vi "PLAN IN FEEDING SCREEN.vi"(6 "LOOP DATA IN":T1, 7 "error IN":errorcluster, 10 "PLAN In":string[][](array[string])) -> (0 "error out":errorcluster, 1 "NO EMPTY CMPLT?":bool, 2 "PLAN Out":string[][](array[string]), 3 "CURRENT PLAN":T2)   [LabVIEW 2017]
uses:
  Controls/LOADING_DISPLAY.ctl
  Controls/Feed_Cyc_Data.ctl
panel:
  # "DOOR NUMBER"
  # "SCANNED CODE"
  # "FEEDER STATUS"
  # "DOOR NUMBER"
  # "SCANNED CODE"
  # "FEEDER STATUS"
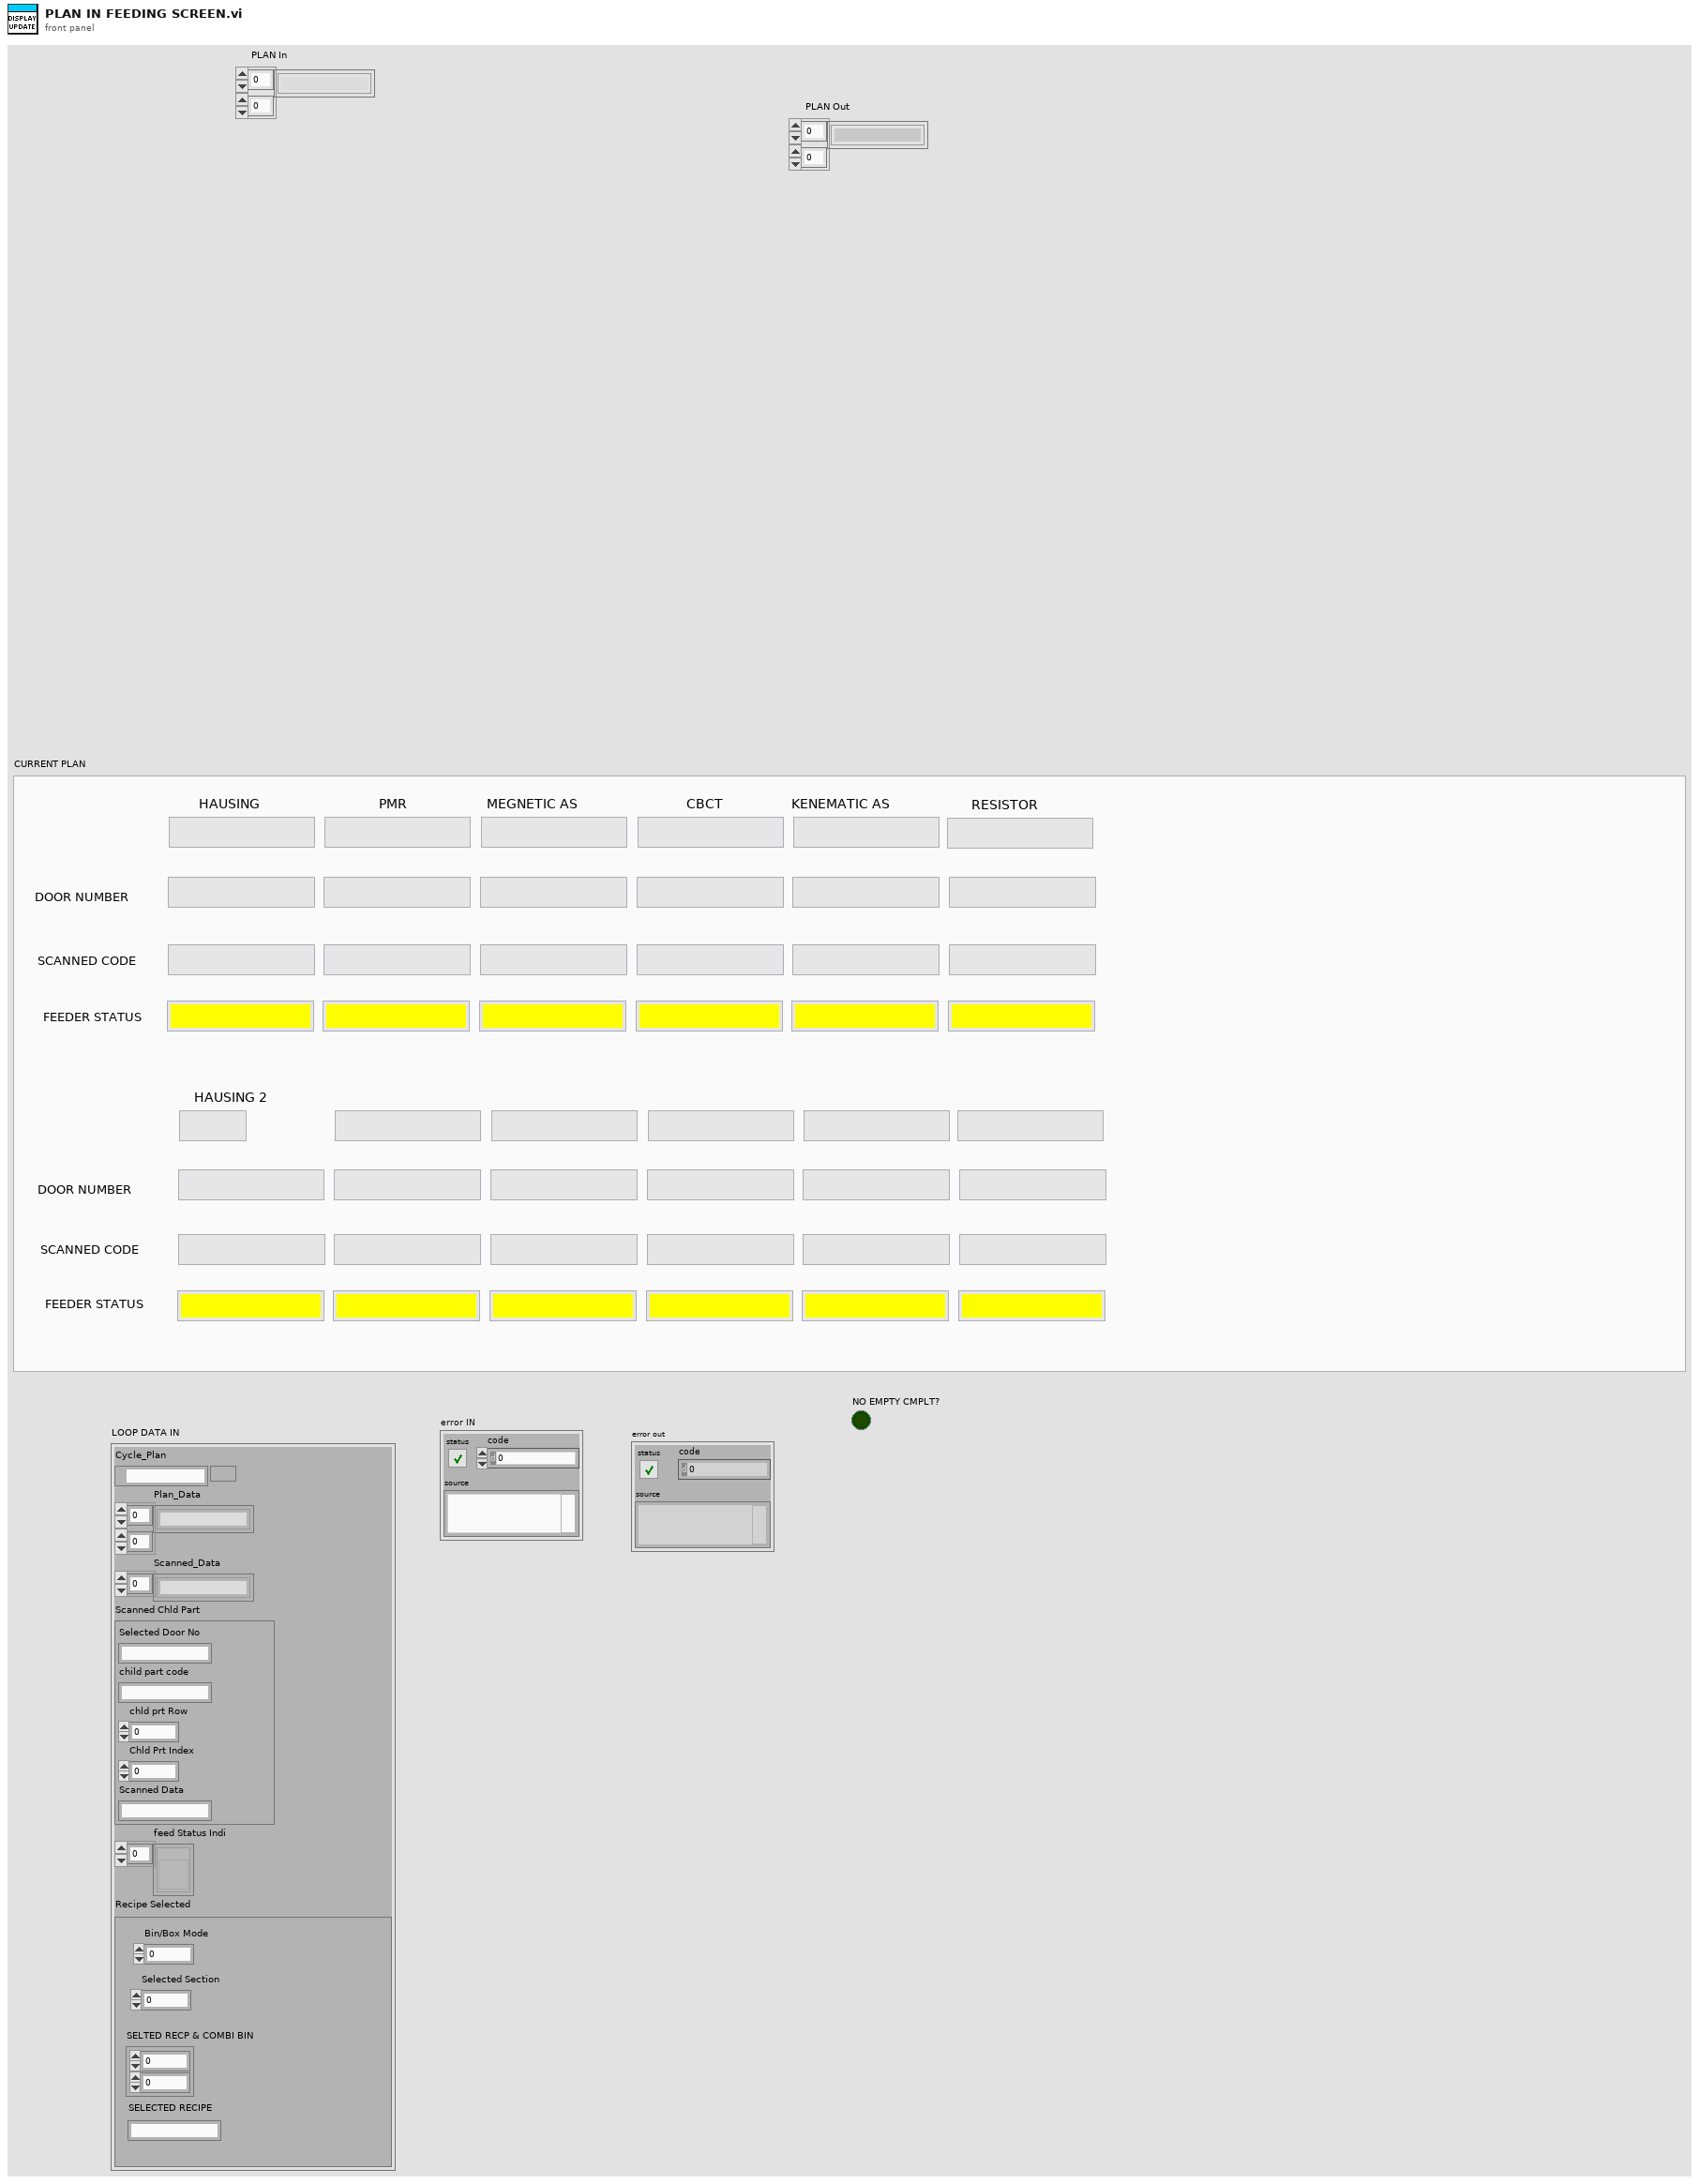
[diagram p1: front panel]
types:
  T1 = typedef "Feed_Cyc_Data.ctl" = cluster{"Cycle_Plan":path, "Plan_Data":string[][], "Scanned_Data":string[], "Scanned Chld Part":cluster{"Selected Door No":string, "child part code":string, "chld prt Row":i32, "Chld Prt Index":i32, "Scanned Data":string}, "feed Status Indi":refnum<vi>[], "Recipe Selected":cluster{"Bin/Box Mode":i32, "Selected Section":i32, "SELTED RECP & COMBI BIN":cluster{i32, i32}, "SELECTED RECIPE":string}}
  T2 = typedef "LOADING_DISPLAY.ctl" = cluster{"HAUSING":string, "PMR":string, "MEGNETIC AS":string, "CBCT":string, "KENEMATIC AS":string, "RESISTOR":string, "HAUSING DOOR":string, "PMR DOOR":string, "MAGNETIC AS DOOR":string, "CBCT DOOR":string, "KINEMATIC AS DOOR":string, "RESISTOR DOOR":string, "HAUSING SCAN QR":string, "PMR SCAN QR":string, "MAGNETIC SCAN QR":string, "CBCT SCAN QR":string, "KINEMATIC SCAN QR":string, "RESISTOR SCAN QR":string, "HAUSING FEED STATUS":string, "PMR FEED STATUS":string, "MAGNETIC AS FEEED STATUS":string, "CBCT FEED STATUS":string, "KINEMATIC AS FEED STATUS":string, "RESISTOR 1 FEED STATUS":string, "HAUSING 2":string, "PMR 2":string, "MEGNETIC AS 2":string, "CBCT 2":string, "KENEMATIC AS 2":string, "RESISTOR 2":string, "HAUSING DOOR 4":string, "PMR DOOR 4":string, "MAGNETIC AS DOOR 4":string, "CBCT DOOR 4":string, "KINEMATIC AS DOOR 4":string, "RESISTOR 1 DOOR 4":string, "HAUSING 2 SCAN QR":string, "PMR 2 SCAN QR":string, "MAGNETIC 2 SCAN QR":string, "CBCT 2 SCAN QR":string, "KINEMATIC 2 SCAN QR":string, "RESISTOR 2 SCAN QR":string, "HAUSING FEED STATUS 2":string, "PMR FEED STATUS 2":string, "MAGNETIC AS FEEED STATUS 2":string, "CBCT FEED STATUS 2":string, "KINEMATIC AS FEED STATUS 2":string, "RESISTOR 1 FEED STATUS 2":string}
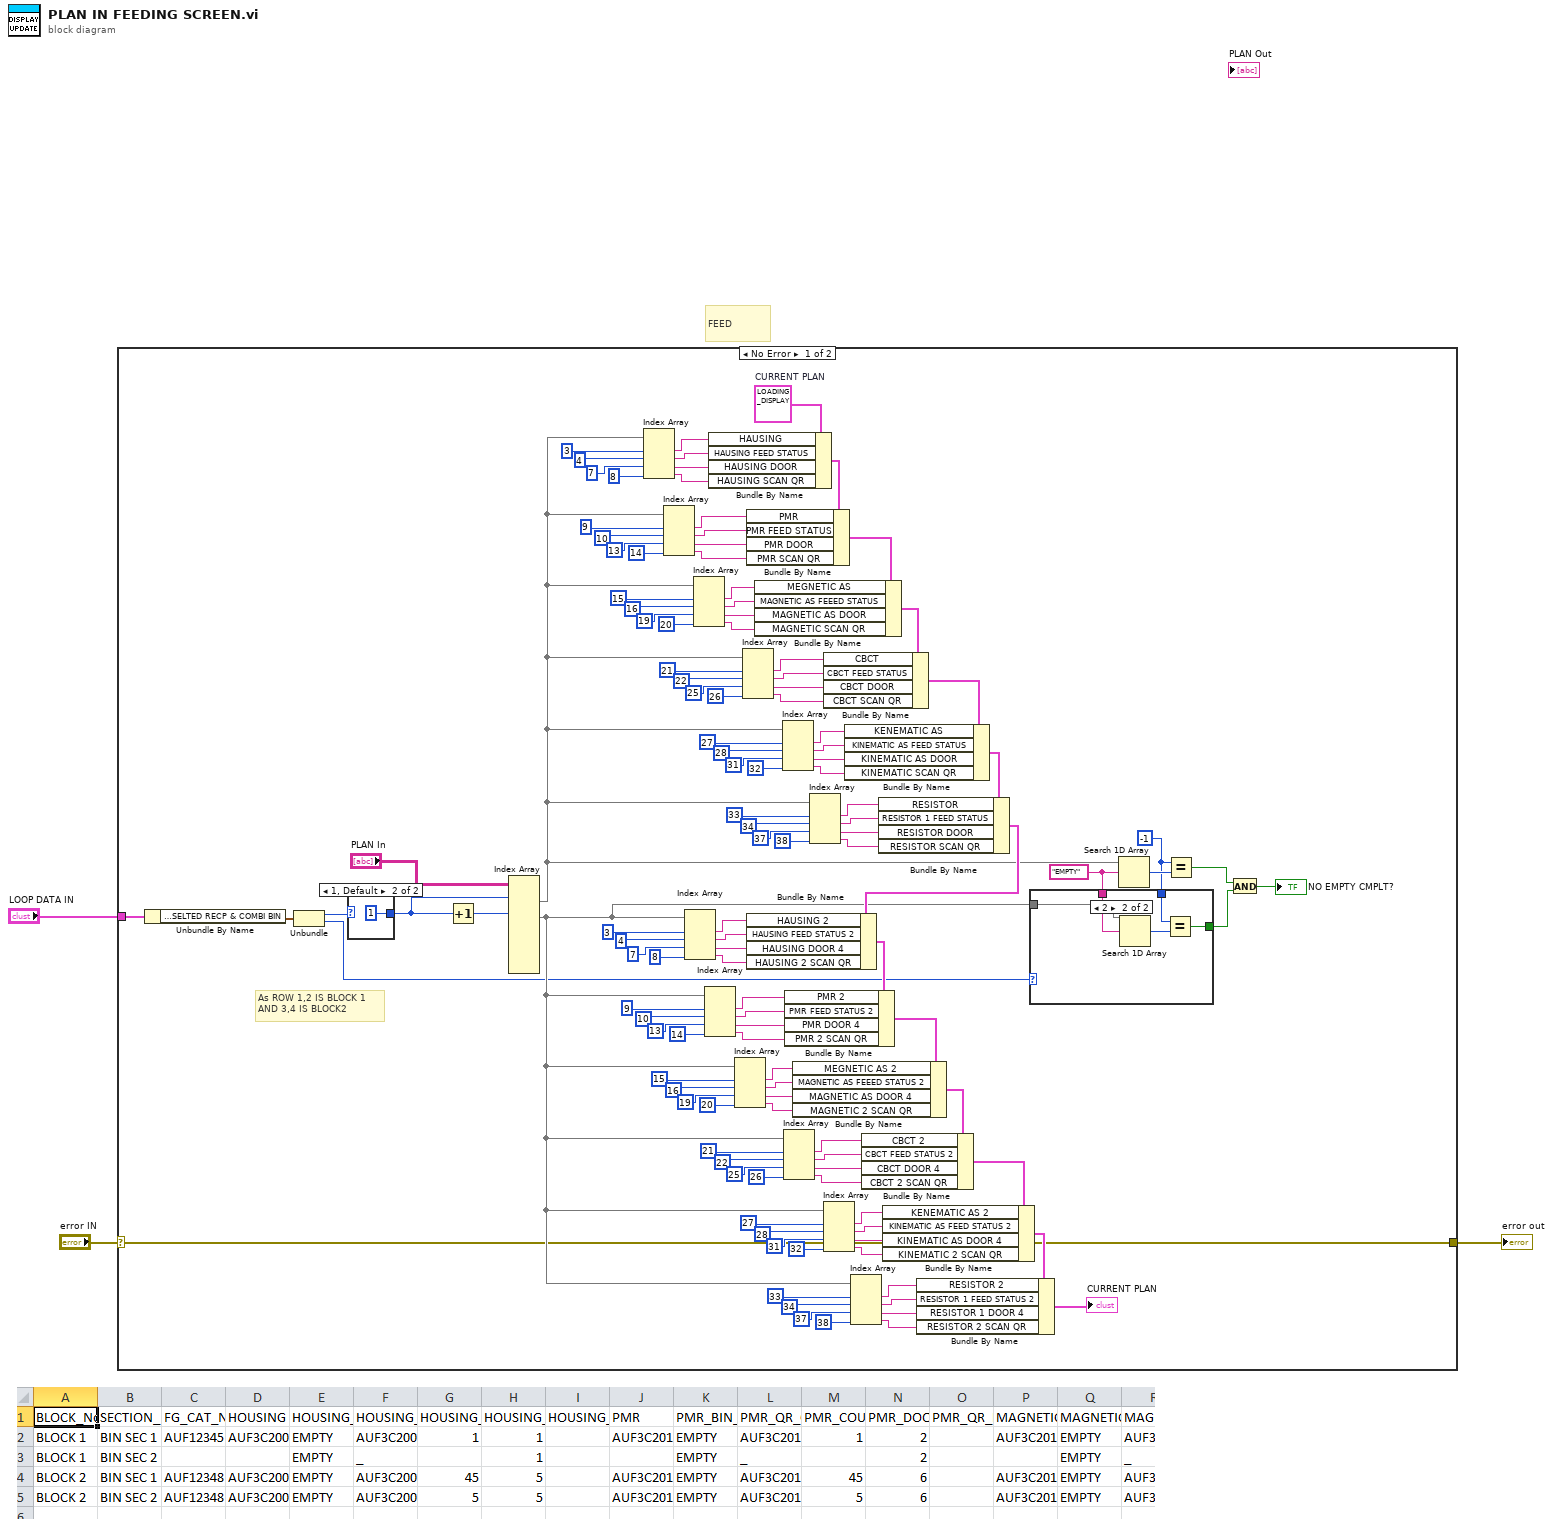
[diagram p0: block diagram]
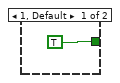
[diagram p2: hidden frame]
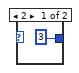
[diagram p3: hidden frame]
diagram:
  # "FEED"
  n1 = case shown="No Error" "error IN" {
    selector: "error IN" -> [w5 w137]
    tunnel: [w5 w137] -> w3
    tunnel: "LOOP DATA IN" -> [w128 _]
    frame No Error {
      w9 = -1
      w11 = "EMPTY"
      w124 = T2 {"HAUSING"="", "PMR"="", "MEGNETIC AS"="", "CBCT"="", "KENEMATIC AS"="", "RESISTOR"="", "HAUSING DOOR"="", "PMR DOOR"="", "MAGNETIC AS DOOR"="", "CBCT DOOR"="", "KINEMATIC AS DOOR"="", "RESISTOR DOOR"="", "HAUSING SCAN QR"="", "PMR SCAN QR"="", "MAGNETIC SCAN QR"="", "CBCT SCAN QR"="", "KINEMATIC SCAN QR"="", "RESISTOR SCAN QR"="", "HAUSING FEED STATUS"="", "PMR FEED STATUS"="", "MAGNETIC AS FEEED STATUS"="", "CBCT FEED STATUS"="", "KINEMATIC AS FEED STATUS"="", "RESISTOR 1 FEED STATUS"="", "HAUSING 2"="", "PMR 2"="", "MEGNETIC AS 2"="", "CBCT 2"="", "KENEMATIC AS 2"="", "RESISTOR 2"="", "HAUSING DOOR 4"="", "PMR DOOR 4"="", "MAGNETIC AS DOOR 4"="", "CBCT DOOR 4"="", "KINEMATIC AS DOOR 4"="", "RESISTOR 1 DOOR 4"="", "HAUSING 2 SCAN QR"="", "PMR 2 SCAN QR"="", "MAGNETIC 2 SCAN QR"="", "CBCT 2 SCAN QR"="", "KINEMATIC 2 SCAN QR"="", "RESISTOR 2 SCAN QR"="", "HAUSING FEED STATUS 2"="", "PMR FEED STATUS 2"="", "MAGNETIC AS FEEED STATUS 2"="", "CBCT FEED STATUS 2"="", "KINEMATIC AS FEED STATUS 2"="", "RESISTOR 1 FEED STATUS 2"=""}  # CURRENT PLAN
      # "As ROW 1,2 IS BLOCK 1 \nAND 3,4 IS BLOCK2"
      n2 = Unbundle By Name(w128) -> ("Recipe Selected.SELTED RECP & COMBI BIN"=w126:cluster{i32, i32})
      n3 = Unbundle(w126) -> (w15:i32, w4:i32)
      n4 = case shown="1, Default" w15 {
        tunnel: [3 1] -> w14
        frame 2 {
        }
        frame 1, Default {
        }
      }
      n5 = Increment(x=w14) -> (x+1=w125:i32)
      n6 = Index Array(array="PLAN In", index (row) #1=w14, index (row) #2=w125) -> (element #1=w13:string[], element #2=w12:string[])  [unwired: 8 in, 3 out]
      n7 = Index Array(array=w13, index #1=3, index #2=4, index #3=7, index #4=8) -> (element #1=w119:string, element #2=w118:string, element #3=w117:string, element #4=w116:string)
      n8 = Index Array(array=w13, index #1=9, index #2=10, index #3=13, index #4=14) -> (element #1=w112:string, element #2=w113:string, element #3=w114:string, element #4=w115:string)
      n9 = Index Array(array=w12, index #1=3, index #2=4, index #3=7, index #4=8) -> (element #1=w22:string, element #2=w23:string, element #3=w24:string, element #4=w25:string)
      n10 = Index Array(array=w13, index #1=15, index #2=16, index #3=19, index #4=20) -> (element #1=w102:string, element #2=w101:string, element #3=w100:string, element #4=w99:string)
      n11 = Index Array(array=w12, index #1=9, index #2=10, index #3=13, index #4=14) -> (element #1=w29:string, element #2=w28:string, element #3=w27:string, element #4=w26:string)
      n12 = Bundle By Name(cluster=w124, "HAUSING"=w119, "HAUSING FEED STATUS"=w118, "HAUSING DOOR"=w117, "HAUSING SCAN QR"=w116) -> (w109:T2)
      n13 = Index Array(array=w12, index #1=15, index #2=16, index #3=19, index #4=20) -> (element #1=w39:string, element #2=w40:string, element #3=w41:string, element #4=w42:string)
      n14 = Index Array(array=w13, index #1=21, index #2=22, index #3=25, index #4=26) -> (element #1=w94:string, element #2=w95:string, element #3=w96:string, element #4=w97:string)
      n15 = Bundle By Name(cluster=w109, "PMR"=w112, "PMR FEED STATUS"=w113, "PMR DOOR"=w114, "PMR SCAN QR"=w115) -> (w98:T2)
      n16 = Bundle By Name(cluster=w98, "MEGNETIC AS"=w102, "MAGNETIC AS FEEED STATUS"=w101, "MAGNETIC AS DOOR"=w100, "MAGNETIC SCAN QR"=w99) -> (w81:T2)
      n17 = Index Array(array=w13, index #1=27, index #2=28, index #3=31, index #4=32) -> (element #1=w85:string, element #2=w84:string, element #3=w83:string, element #4=w82:string)
      n18 = Index Array(array=w12, index #1=21, index #2=22, index #3=25, index #4=26) -> (element #1=w47:string, element #2=w46:string, element #3=w45:string, element #4=w44:string)
      n19 = Index Array(array=w13, index #1=33, index #2=34, index #3=37, index #4=38) -> (element #1=w76:string, element #2=w77:string, element #3=w78:string, element #4=w79:string)
      n20 = Bundle By Name(cluster=w81, "CBCT"=w94, "CBCT FEED STATUS"=w95, "CBCT DOOR"=w96, "CBCT SCAN QR"=w97) -> (w80:T2)
      n21 = Index Array(array=w12, index #1=27, index #2=28, index #3=31, index #4=32) -> (element #1=w56:string, element #2=w57:string, element #3=w58:string, element #4=w59:string)
      n22 = Bundle By Name(cluster=w80, "KENEMATIC AS"=w85, "KINEMATIC AS FEED STATUS"=w84, "KINEMATIC AS DOOR"=w83, "KINEMATIC SCAN QR"=w82) -> (w71:T2)
      n23 = Index Array(array=w12, index #1=33, index #2=34, index #3=37, index #4=38) -> (element #1=w65:string, element #2=w64:string, element #3=w63:string, element #4=w62:string)
      n24 = Bundle By Name(cluster=w71, "RESISTOR"=w76, "RESISTOR 1 FEED STATUS"=w77, "RESISTOR DOOR"=w78, "RESISTOR SCAN QR"=w79) -> (w17:T2)
      n25 = Bundle By Name(cluster=w17, "HAUSING 2"=w22, "HAUSING FEED STATUS 2"=w23, "HAUSING DOOR 4"=w24, "HAUSING 2 SCAN QR"=w25) -> (w32:T2)
      n26 = Bundle By Name(cluster=w32, "PMR 2"=w29, "PMR FEED STATUS 2"=w28, "PMR DOOR 4"=w27, "PMR 2 SCAN QR"=w26) -> (w43:T2)
      n27 = Bundle By Name(cluster=w43, "MEGNETIC AS 2"=w39, "MAGNETIC AS FEEED STATUS 2"=w40, "MAGNETIC AS DOOR 4"=w41, "MAGNETIC 2 SCAN QR"=w42) -> (w60:T2)
      n28 = Bundle By Name(cluster=w60, "CBCT 2"=w47, "CBCT FEED STATUS 2"=w46, "CBCT DOOR 4"=w45, "CBCT 2 SCAN QR"=w44) -> (w61:T2)
      n29 = Bundle By Name(cluster=w61, "KENEMATIC AS 2"=w56, "KINEMATIC AS FEED STATUS 2"=w57, "KINEMATIC AS DOOR 4"=w58, "KINEMATIC 2 SCAN QR"=w59) -> (w70:T2)
      n30 = Bundle By Name(cluster=w70, "RESISTOR 2"=w65, "RESISTOR 1 FEED STATUS 2"=w64, "RESISTOR 1 DOOR 4"=w63, "RESISTOR 2 SCAN QR"=w62) -> (→"CURRENT PLAN":T2)
      n31 = case shown="2" w4 {
        tunnel: w12 -> [_ w134]
        tunnel: w11 -> [_ w133]
        tunnel: w9 -> [_ w131]
        tunnel: [TRUE w130] -> w6
        frame 1, Default {
        }
        frame 2 {
          n32 = Search 1D Array(1D array=w134, element=w133) -> (index of element=w132:i32)  [unwired: 1 in]
          n33 = Equal?(x=w131, y=w132) -> (x = y?=w130:bool)
        }
      }
      n34 = Search 1D Array(1D array=w13, element=w11) -> (index of element=w10:i32)  [unwired: 1 in]
      n35 = Equal?(x=w9, y=w10) -> (x = y?=w8:bool)
      n36 = And(x=w8, y=w6) -> (x .and. y?=→"NO EMPTY CMPLT?":bool)
    }
    frame Error {
    }
  }
  "error out" <- w3
